vi "CheckSavedFile.vi"(7 "Name":string="Main.py", 8 "error in (no error)":errorcluster, 9 "Console in":string, 10 "All Code":string, 11 "VISA in":refnum<visa-resource-name>) -> (0 "error out":errorcluster, 1 "Console Out":string, 2 "Success?":bool, 3 "VISA out":refnum<visa-resource-name>, 4 "Saved Contents":string)   [LabVIEW 2016]
panel:
  in  "Reply":string
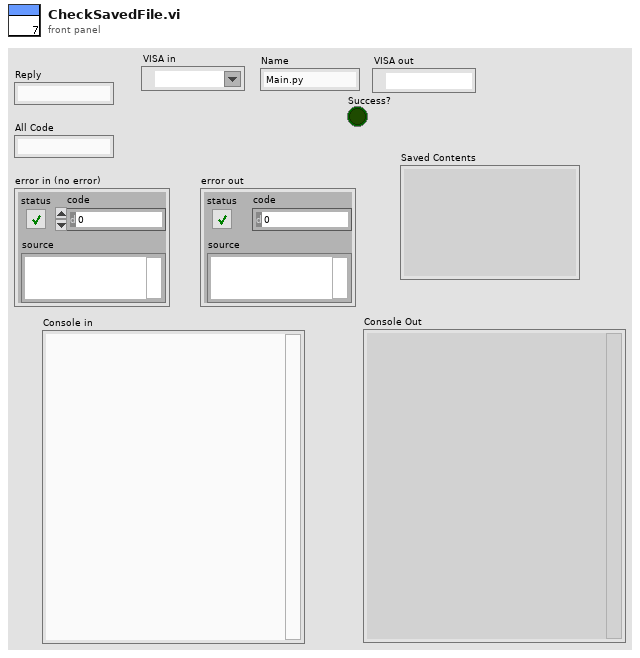
[diagram p1: front panel]
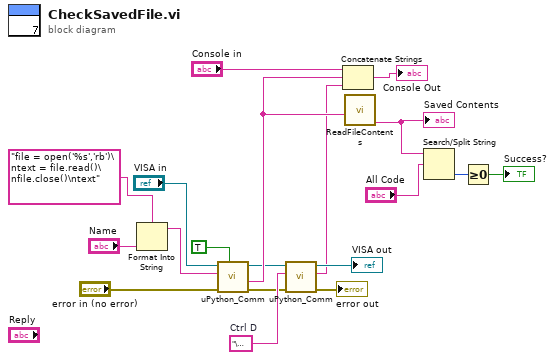
[diagram p0: block diagram]
diagram:
  w4 = "\u0004"  # Ctrl D
  n1 = Format Into String(format string="file = open('%s','rb')\ntext = file.read()\nfile.close()\ntext" ("write buffer"), "Name") -> (resulting string=w19:string)  [unwired: 2 in, 1 out]
  n2 = call "uPython_Comm.vi"("Wait for Reply?"=TRUE, "error in (no error)"="error in (no error)", "Script"=w19, "VISA Refnum in"="VISA in") -> ("error out"=w3:errorcluster, "Console Out"=w9:string, "VISA out"=w6:refnum<visa-resource-name>)  [unwired: 3 in, 2 out]
  n3 = call "uPython_Comm.vi"("error in (no error)"=w3, "Script"=w4, "VISA Refnum in"=w6) -> ("error out"=→"error out":errorcluster, "Buffer"=w1:string, "VISA out"=→"VISA out":refnum<visa-resource-name>)  [unwired: 4 in, 2 out]
  n4 = Concatenate Strings("Console in", w9, w1) -> (→"Console Out":string)
  n5 = call "ReadFileContents.vi"("Console"=w9) -> ("File Contents"=w8:string)  [unwired: 9 in, 1 out]
  "Saved Contents" <- w8
  n6 = Search/Split String(string=w8, search string/char (-)="All Code") -> (offset of match=w13:i32)  [unwired: 1 in, 2 out]
  n7 = Greater Or Equal To 0?(x=w13) -> (x >= 0?=→"Success?":bool)
